vi "MSControl_main.vi"() -> ()   [LabVIEW 2017]
doc: "this is the start vi forMSControl program"
uses:
  Classes/StatusLog/StatusLog.lvclass
  Classes/PrepLineObject/PrepLineObject.lvclass
  Classes/Flags/flag.lvclass
  Classes/Plots/Plots.lvclass
  Classes/Standard/Standard.lvclass
  Classes/Spectrometer/Spectrometer.lvclass
  Classes/Analysis/Analysis.lvclass
  Classes/Instrument/instrument.lvclass
  Classes/MagFieldTable/MagFieldTable.lvclass
  Classes/Pipette/Pipette.lvclass
  Classes/Message/Message.lvclass
  global variables.vi
  <vilib>/Utility/config.llb/Read Key (U32).vi
  <vilib>/Utility/config.llb/Read Key (Path).vi
  <vilib>/Utility/config.llb/Read Key (String).vi
  <vilib>/Utility/config.llb/NI_LVConfig.lvlib
panel:
  in  "setup button":bool
  in  "start button":bool
  out "status string":string
  in  "error in (no error)":errorcluster
  out "error out":errorcluster
  # "MS Control"
  # "v20171231"
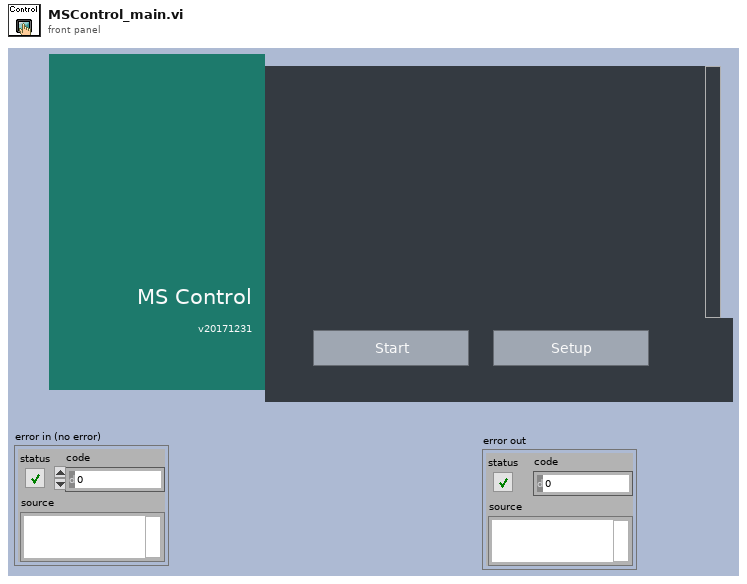
[diagram p1: front panel]
types:
  T1 = cluster{"log identifier":string, "active?":bool}[]
  T2 = cluster{"name":string, "inst-type":string, "class path":path, "class-name":string}[]
  T3 = cluster{"name":string, "class-name":string, "class path":path, "inst-type":string}
  T4 = cluster{"event name":enum16{"SwitchUpdate", "SysChkUpdate", "ScriptMessageUpdate"}}
  T5 = typedef "NI_LVConfig.lvlib/Config Data RefNum.ctl" = refnum<k1>
  T6 = cluster{"name":string, "class-name":string, "class path":path, "inst-type":string}[]
  T7 = cluster{"name":string, "inst-type":string, "class path":path, "class-name":string}
  T8 = typedef "Semaphore RefNum" = refnum<k1>
  T9 = enum32{"Invalid", "Standard", "Closed", "Hidden", "Minimized", "Maximized"}
  T10 = enum16{"Left Button", "Center Button", "Right Button", "Window Close"}
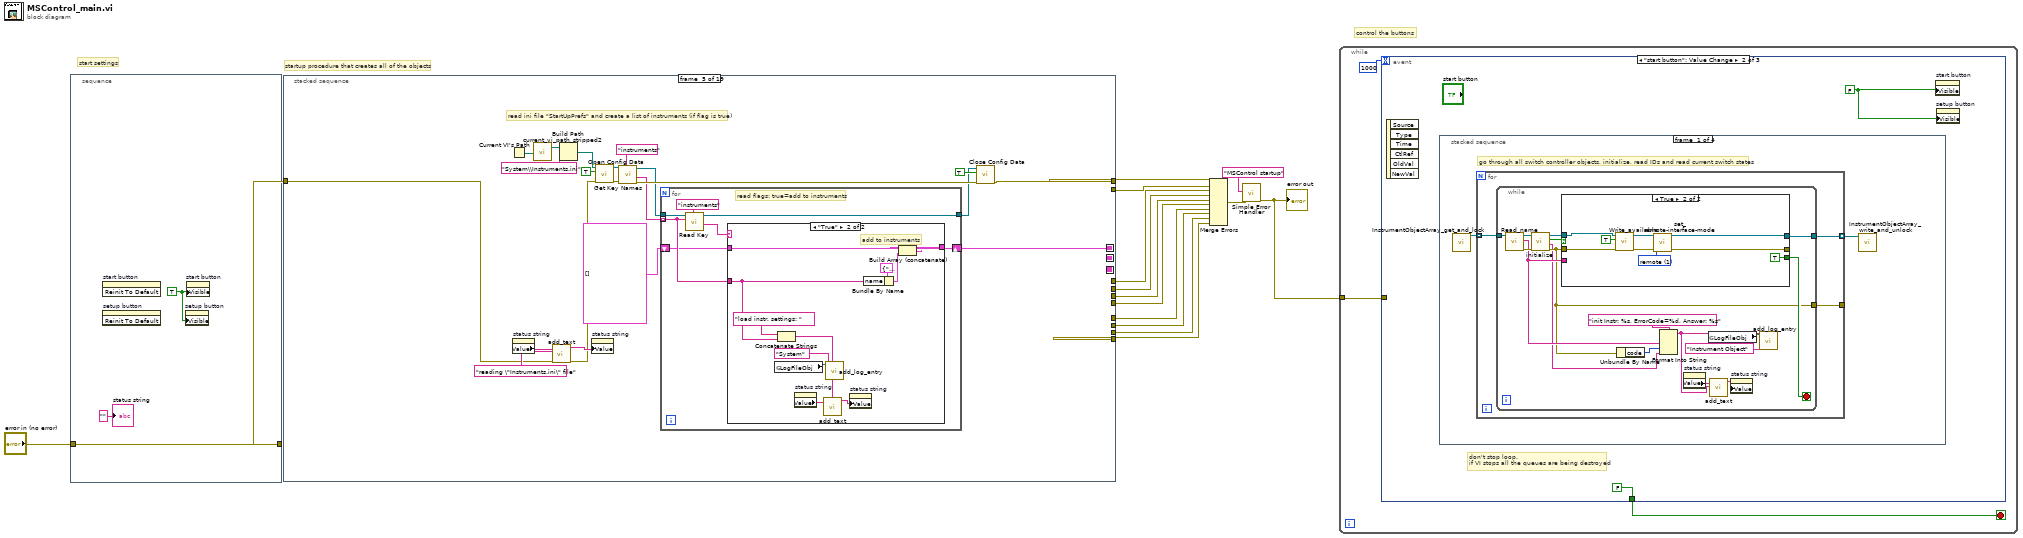
[diagram p0: block diagram]
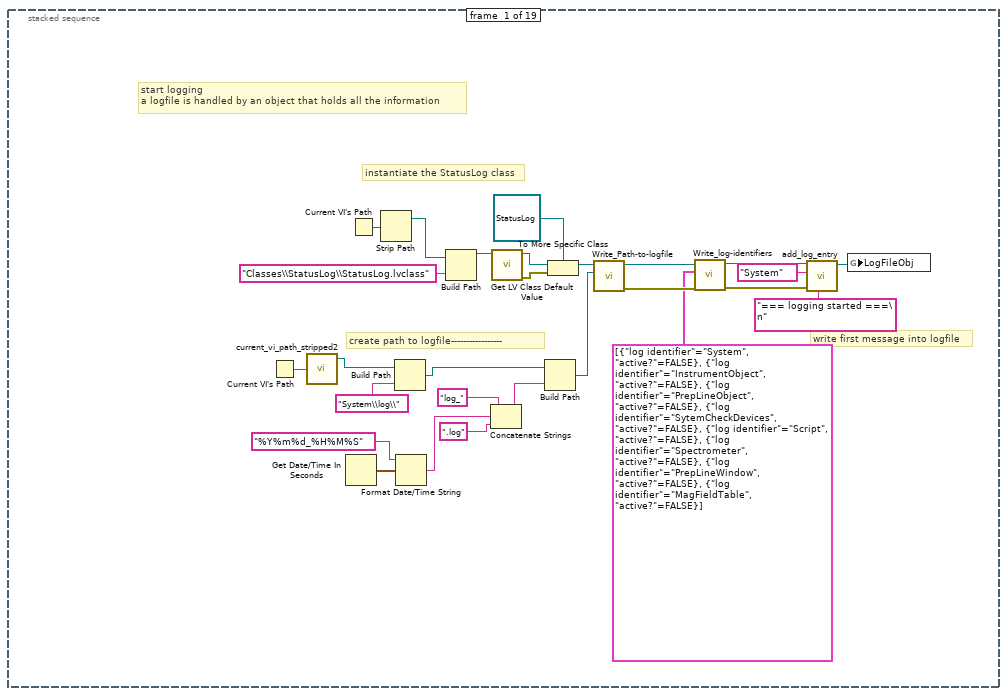
[diagram p2: hidden frame]
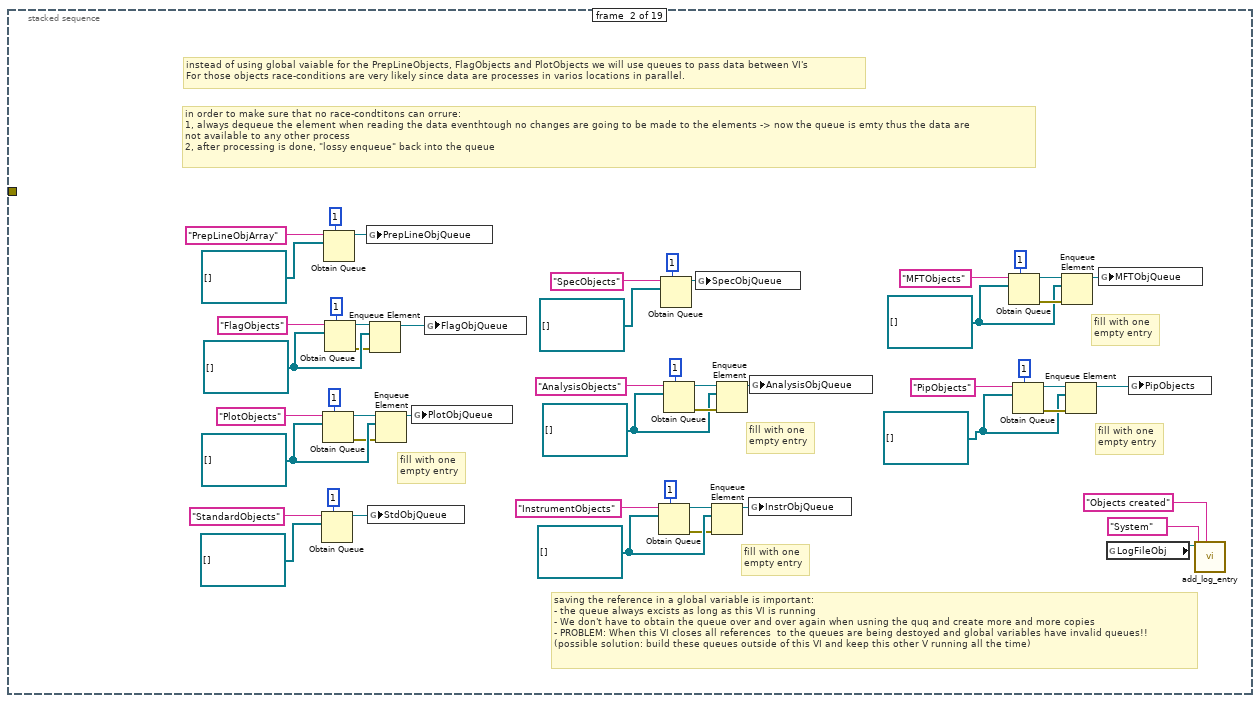
[diagram p3: hidden frame]
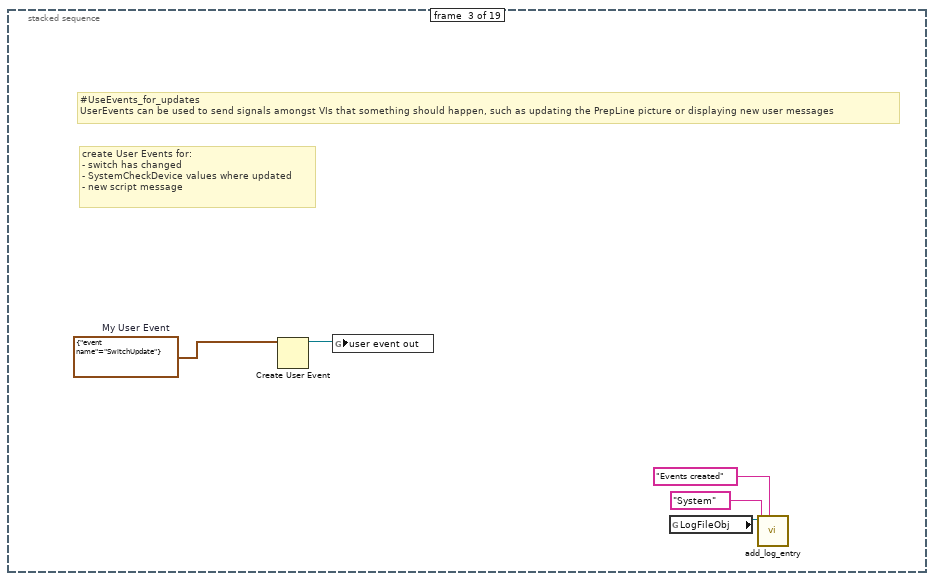
[diagram p4: hidden frame]
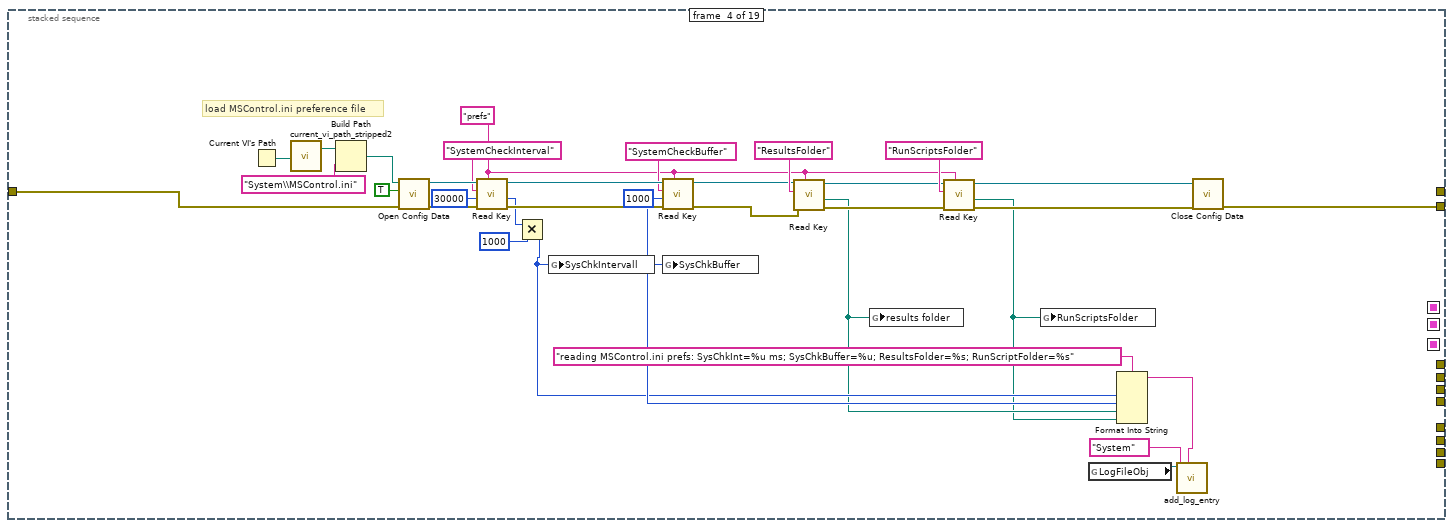
[diagram p5: hidden frame]
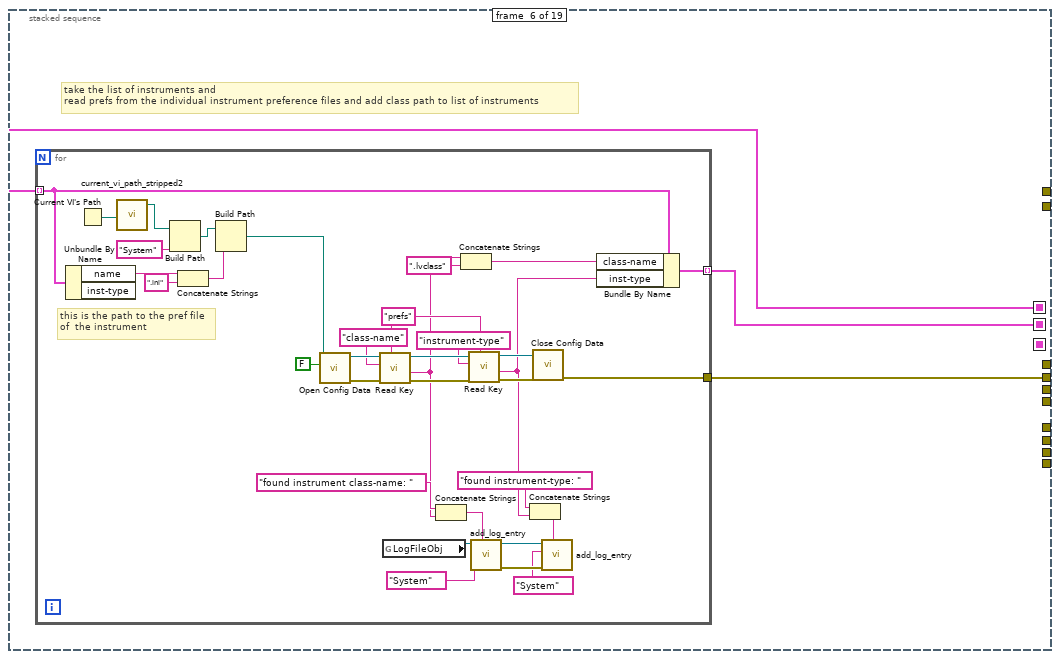
[diagram p7: hidden frame]
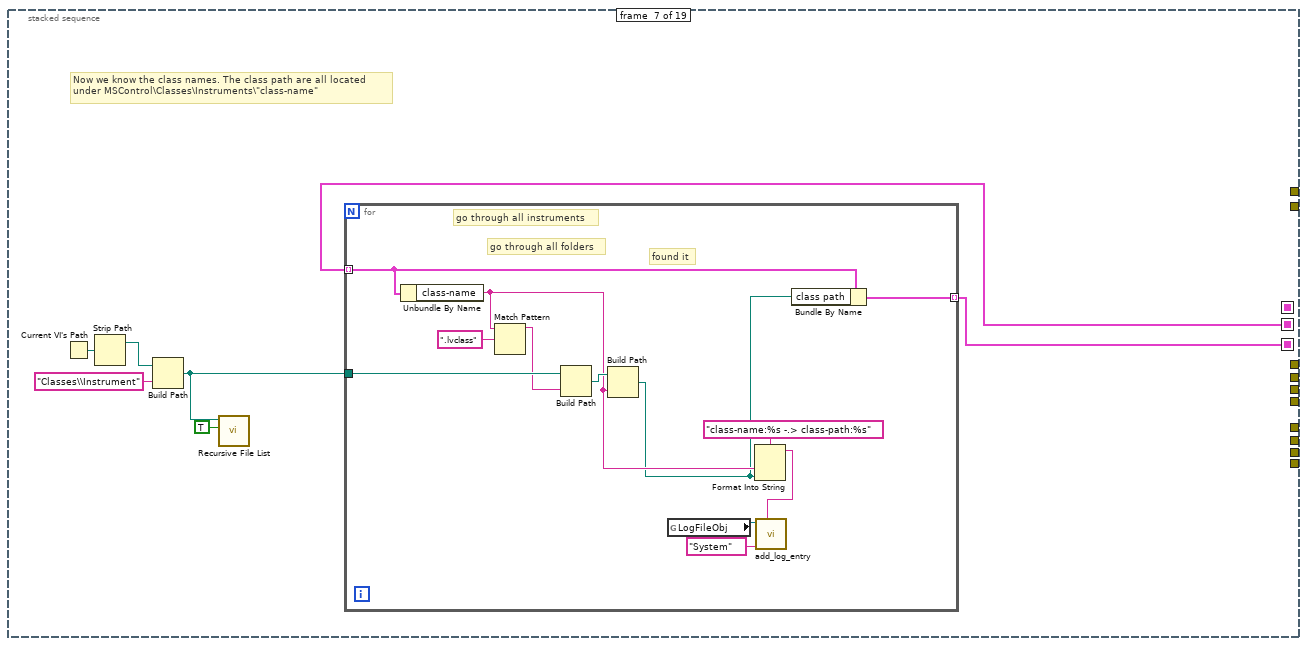
[diagram p8: hidden frame]
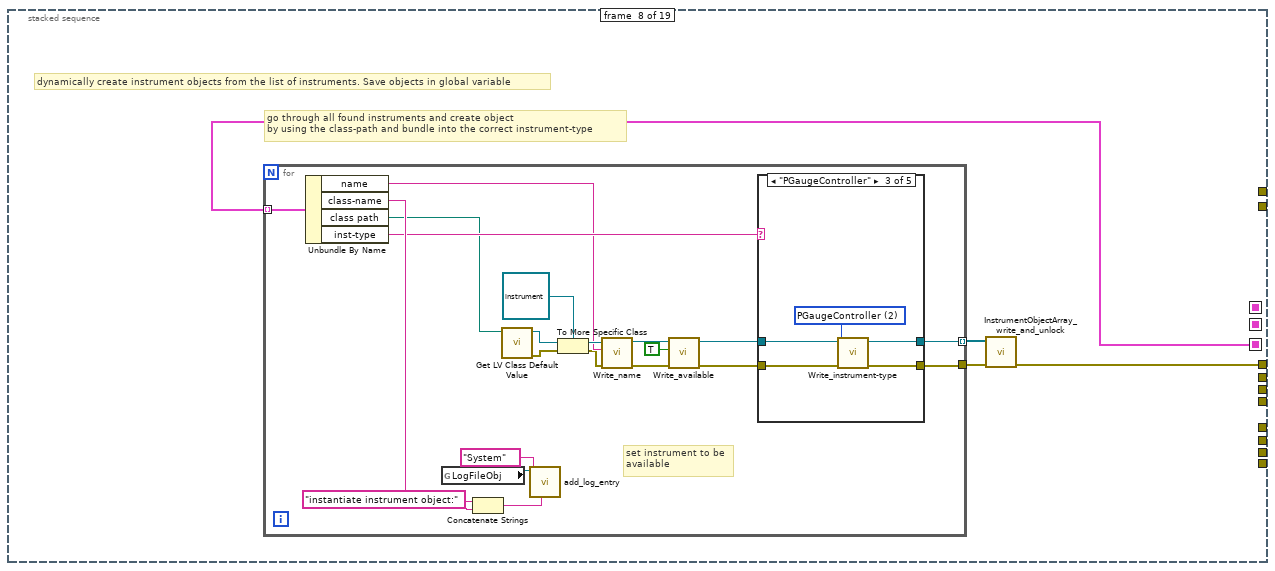
[diagram p9: hidden frame]
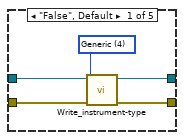
[diagram p10: hidden frame]
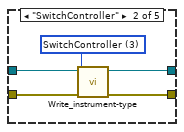
[diagram p11: hidden frame]
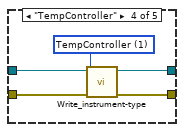
[diagram p12: hidden frame]
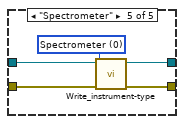
[diagram p13: hidden frame]
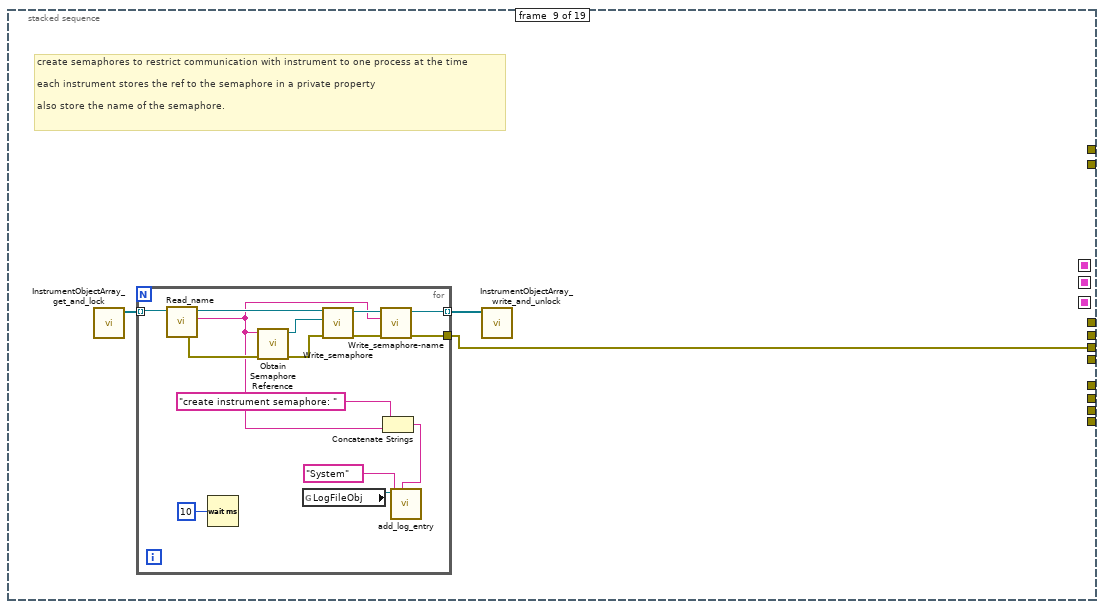
[diagram p14: hidden frame]
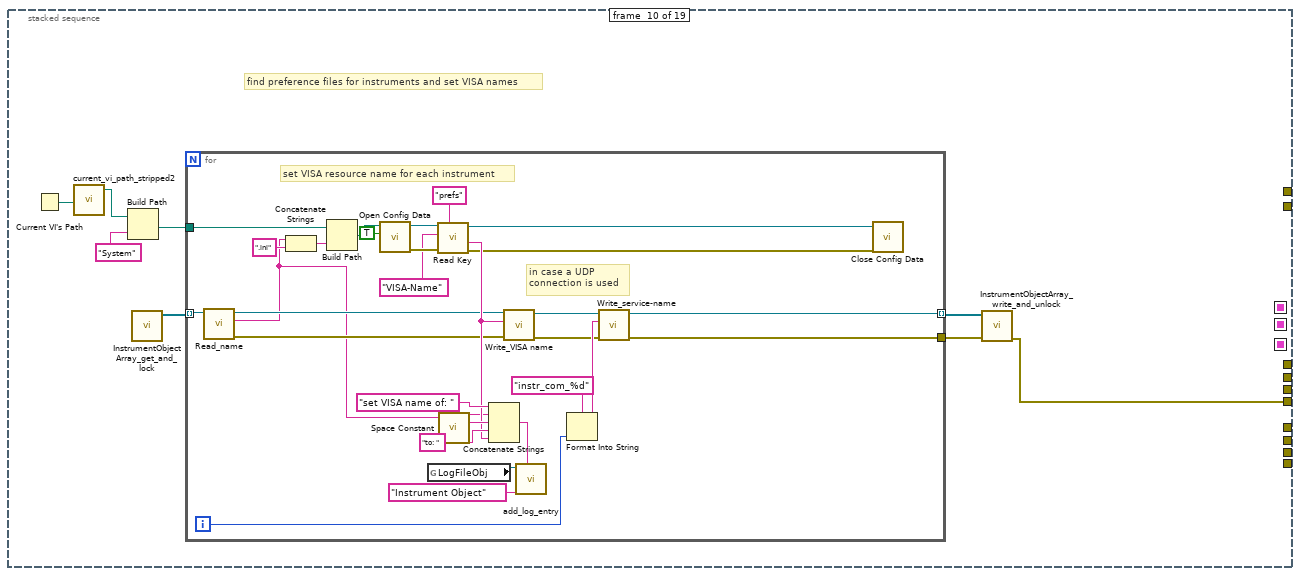
[diagram p15: hidden frame]
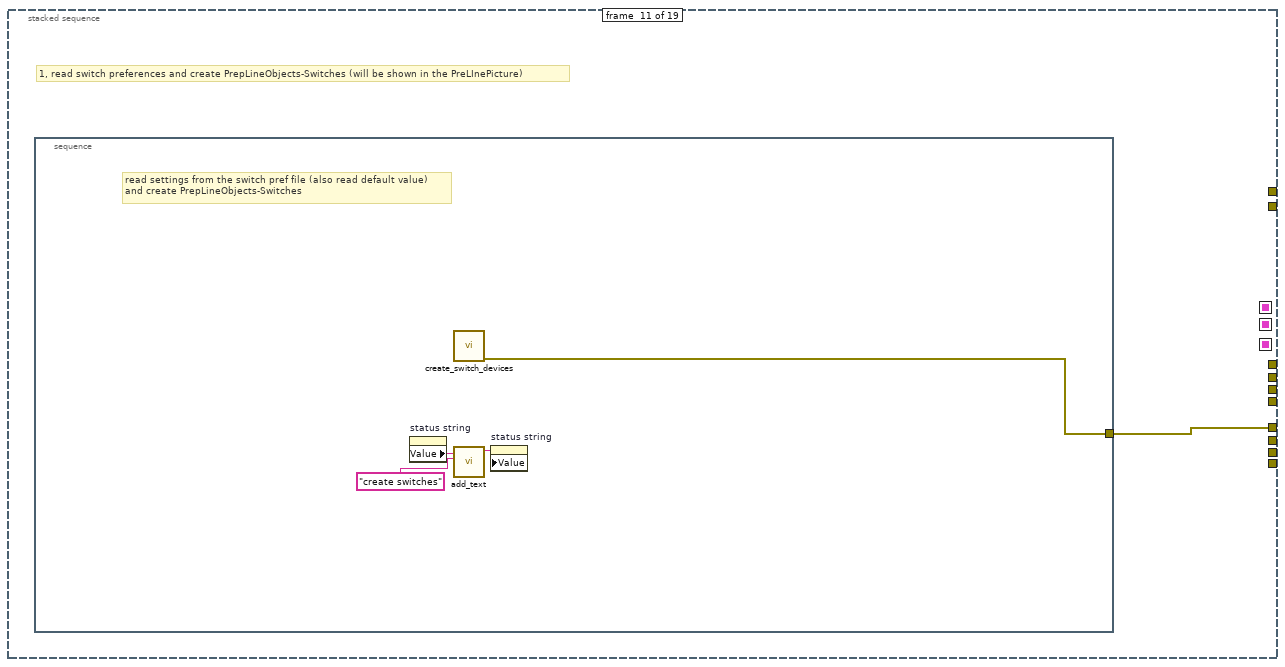
[diagram p16: hidden frame]
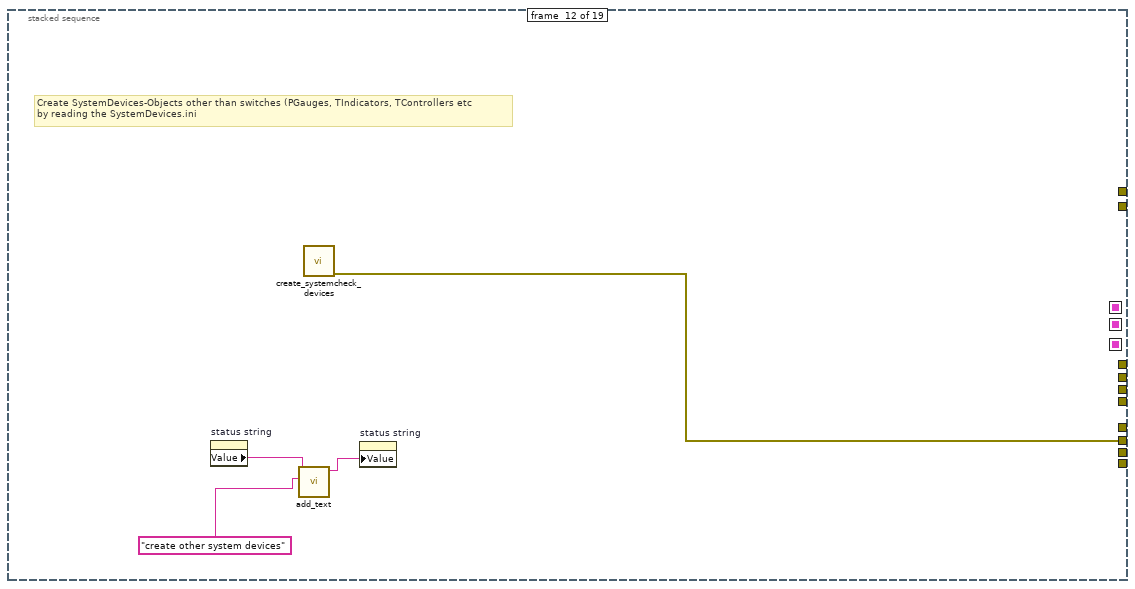
[diagram p17: hidden frame]
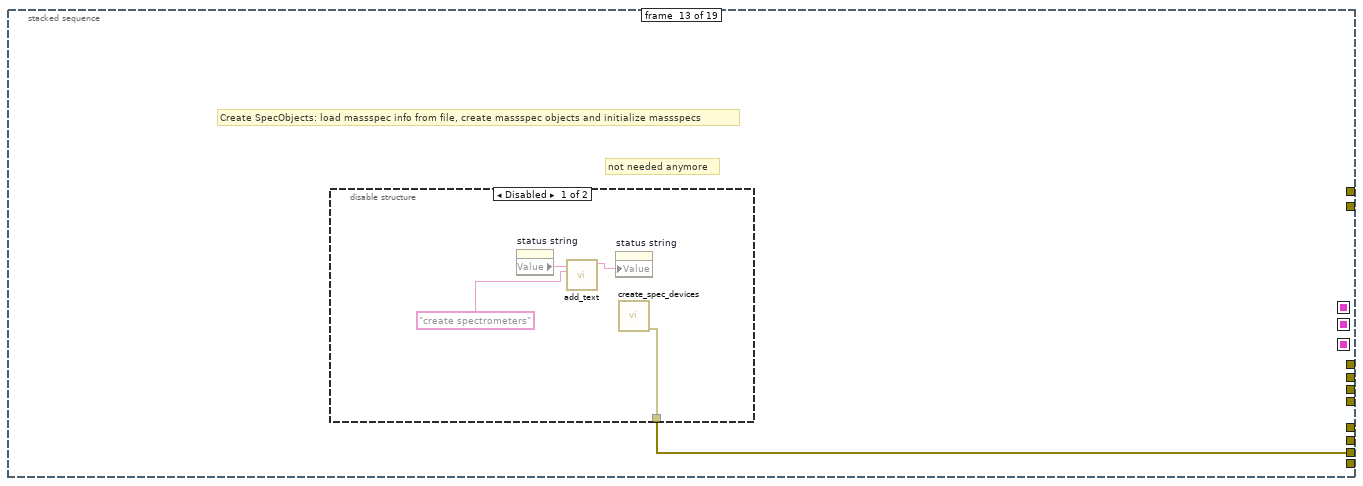
[diagram p18: hidden frame]
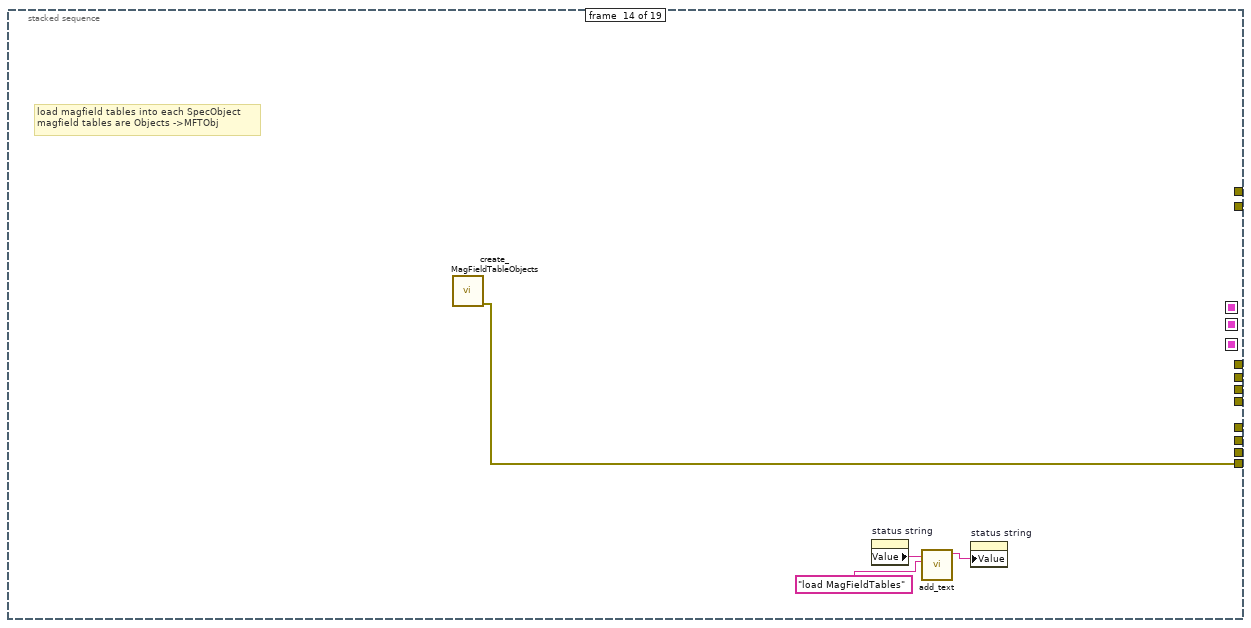
[diagram p20: hidden frame]
diagram:
  # "start settings"
  # "startup procedure that creates all of the objects"
  # "control the buttons"
  n1 = stacked-sequence {
    tunnel: [w17] -> w14
    tunnel: "error in (no error)" -> [w17]
    frame #0 {
      w16 = TRUE ("Visible")
      n2 = invoke on="start button" class="Bool (strict)" method="Reinit To Default"() -> ()  [unwired: 3 in, 3 out]
      n3 = invoke on="setup button" class="Bool (strict)" method="Reinit To Default"() -> ()  [unwired: 3 in, 3 out]
      n4 = property on="setup button" class="Bool (strict)"("Visible"=w16) -> ()  [unwired: 2 in, 2 out]
      n5 = property on="start button" class="Bool (strict)"("Visible"=w16) -> ()  [unwired: 2 in, 2 out]
      "status string" <- "" ("status string")
    }
  }
  n6 = stacked-sequence {
    seq-local: [_ _ _ _ w139 _ _ _ _ _ _ _ _ _ _ _ _ _ _] -> [_ _ _ _ _ w178 _ _ _ _ _ _ _ _ _ _ _ _ _]
    seq-local: [_ _ _ _ _ w177 _ _ _ _ _ _ _ _ _ _ _ _ _] -> [_ _ _ _ _ _ w218 _ _ _ _ _ _ _ _ _ _ _ _]
    seq-local: [_ _ _ _ _ _ w217 _ _ _ _ _ _ _ _ _ _ _ _] -> [_ _ _ _ _ _ _ w235 _ _ _ _ _ _ _ _ _ _ _]
    tunnel: w14 -> [_ _ _ w122 w141 _ _ _ _ _ _ _ _ _ _ _ _ _ _]
    tunnel: [_ _ _ _ w150 _ _ _ _ _ _ _ _ _ _ _ _ _ _] -> w13
    tunnel: [_ _ _ w121 _ _ _ _ _ _ _ _ _ _ _ _ _ _ _] -> w12
    tunnel: [_ _ _ _ _ w176 _ _ _ _ _ _ _ _ _ _ _ _ _] -> w10
    tunnel: [_ _ _ _ _ _ _ w232 _ _ _ _ _ _ _ _ _ _ _] -> w11
    tunnel: [_ _ _ _ _ _ _ _ w284 _ _ _ _ _ _ _ _ _ _] -> w9
    tunnel: [_ _ _ _ _ _ _ _ _ w300 _ _ _ _ _ _ _ _ _] -> w8
    tunnel: [_ _ _ _ _ _ _ _ _ _ w337 _ _ _ _ _ _ _ _] -> w7
    tunnel: [_ _ _ _ _ _ _ _ _ _ _ w345 _ _ _ _ _ _ _] -> w6
    tunnel: [_ _ _ _ _ _ _ _ _ _ _ _ w346 _ _ _ _ _ _] -> w3
    tunnel: [_ _ _ _ _ _ _ _ _ _ _ _ _ w351 _ _ _ _ _] -> w2
    frame #0 {
      # "write first message into logfile"
      # "create path to logfile-----------------"
      # "instantiate the StatusLog class"
      # "start logging\na logfile is handled by an object that holds all the information"
      n7 = Current VI's Path() -> (path=w20:path)
      n8 = call "current_vi_path_stripped2.vi"("current VI Path"=w20) -> ("current VI Path stripped out"=w19:path)  [unwired: 3 in, 1 out]
      n9 = Get Date/Time In Seconds() -> (seconds since 1Jan1904=w37:timestamp)
      n10 = Current VI's Path() -> (path=w22:path)
      n11 = Strip Path(path=w22) -> (stripped path=w21:path)  [unwired: 1 out]
      n12 = Build Path(base path=w19, name or relative path="System\\log\\") -> (appended path=w38:path)
      n13 = Format Date/Time String(time format string (%c)="%Y%m%d_%H%M%S", seconds (now)=w37) -> (date/time string=w33:string)  [unwired: 1 in]
      n14 = Build Path(base path=w21, name or relative path="Classes\\StatusLog\\StatusLog.lvclass") -> (appended path=w41:path)
      n15 = Concatenate Strings("log_" ("string"), w33, ".log" ("string")) -> (w35:string)
      n16 = call <vilib>:"Get LV Class Default Value.vi"("class path"=w41) -> ("error out"=w43:errorcluster, "object"=w44:refnum<class>)  [unwired: 1 in, 8 out]
      n17 = Build Path(base path=w38, name or relative path=w35) -> (appended path=w34:path)
      n18 = To More Specific Class(target class=refnum<class "StatusLog.lvclass"> refnum ("StatusLog.lvclass"), reference=w44, error in=w43) -> (specific class reference=w39:refnum<class "StatusLog.lvclass">)  [unwired: 1 out]
      n19 = call-dynamic "Write_Path-to-logfile.vi"("Path to logfile"=w34, "StatusLog in"=w39) -> ("error out"=w26:errorcluster, "StatusLog out"=w28:refnum<class "StatusLog.lvclass">)  [unwired: 8 in]
      n20 = call-dynamic "Write_log-identifiers.vi"("error in (no error)"=w26, "log identifiers"=T1 [{"log identifier"="System", "active?"=FALSE}, {"log identifier"="InstrumentObject", "active?"=FALSE}, {"log identifier"="PrepLineObject", "active?"=FALSE}, {"log identifier"="SytemCheckDevices", "active?"=FALSE}, {"log identifier"="Script", "active?"=FALSE}, {"log identifier"="Spectrometer", "active?"=FALSE}, {"log identifier"="PrepLineWindow", "active?"=FALSE}, {"log identifier"="MagFieldTable", "active?"=FALSE}], "StatusLog in"=w28) -> ("error out"=w25:errorcluster, "StatusLog out"=w27:refnum<class "StatusLog.lvclass">)  [unwired: 7 in]
      n21 = call-dynamic "add_log_entry.vi"("new entry"="=== logging started ===\n", "error in (no error)"=w25, "log identifiers"="System", "StatusLog in"=w27) -> ("StatusLog out"=w29:refnum<class "StatusLog.lvclass">)  [unwired: 4 in, 1 out]
      n22 = global write "global variables.vi" "LogFileObj"(w29) -> ()
    }
    frame #1 {
      w49 = refnum<class "Pipette.lvclass">[] [] ("PlotObjArray")
      w63 = refnum<class "MagFieldTable.lvclass">[] [] ("PlotObjArray")
      w66 = refnum<class "instrument.lvclass">[] [] ("PlotObjArray")
      w75 = refnum<class "Analysis.lvclass">[] [] ("PlotObjArray")
      w79 = refnum<class "Plots.lvclass">[] [] ("PlotObjArray")
      w57 = refnum<class "flag.lvclass">[] [] ("FlagObjArray")
      # "fill with one\nempty entry"
      # "fill with one\nempty entry"
      # "fill with one\nempty entry"
      # "fill with one\nempty entry"
      # "fill with one\nempty entry"
      # "saving the reference in a global variable is important:\n- the queue always excists as long as this VI is running\n- We don't have to obtain the queue over and over again when usning the quq and create more and more copies\n- PROBLEM: When this VI closes all references  to the queues are being destoyed and global variables have invalid queues!!\n(possible solution: build these queues outside of this VI and keep this other V running all the time)"
      # "in order to make sure that no race-condtitons can orrure:\n1, always dequeue the element when reading the data eventhtough no changes are going to be made to the elements -> now the queue is emty thus the data are\nnot available to any other process\n2, after processing is done, \"lossy enqueue\" back into the queue"
      # "instead of using global vaiable for the PrepLineObjects, FlagObjects and PlotObjects we will use queues to pass data between VI's\nFor those objects race-conditions are very likely since data are processes in varios locations in parallel."
      n23 = Obtain Queue(max queue size (-1, unlimited)=1, name (unnamed)="StandardObjects", element data type=refnum<class "Standard.lvclass">[] [] ("PlotObjArray")) -> (queue out=w85:refnum<queue>)  [unwired: 2 in, 2 out]
      n24 = Obtain Queue(max queue size (-1, unlimited)=1, name (unnamed)="PlotObjects", element data type=w79) -> (queue out=w80:refnum<queue>, error out=w77:errorcluster)  [unwired: 2 in, 1 out]
      n25 = Obtain Queue(max queue size (-1, unlimited)=1, name (unnamed)="PrepLineObjArray", element data type=refnum<class "PrepLineObject.lvclass">[] [] ("PrepLineObjArray")) -> (queue out=w89:refnum<queue>)  [unwired: 2 in, 2 out]
      n26 = Obtain Queue(max queue size (-1, unlimited)=1, name (unnamed)="FlagObjects", element data type=w57) -> (queue out=w58:refnum<queue>, error out=w56:errorcluster)  [unwired: 2 in, 1 out]
      n27 = global write "global variables.vi" "PrepLineObjQueue"(w89) -> ()
      n28 = global write "global variables.vi" "StdObjQueue"(w85) -> ()
      n29 = Enqueue Element(queue=w58, element=w57, error in (no error)=w56) -> (queue out=w55:refnum<queue>)  [unwired: 1 in, 2 out]
      n30 = Enqueue Element(queue=w80, element=w79, error in (no error)=w77) -> (queue out=w78:refnum<queue>)  [unwired: 1 in, 2 out]
      n31 = global write "global variables.vi" "PlotObjQueue"(w78) -> ()
      n32 = global write "global variables.vi" "FlagObjQueue"(w55) -> ()
      n33 = Obtain Queue(max queue size (-1, unlimited)=1, name (unnamed)="InstrumentObjects", element data type=w66) -> (queue out=w67:refnum<queue>, error out=w65:errorcluster)  [unwired: 2 in, 1 out]
      n34 = Obtain Queue(max queue size (-1, unlimited)=1, name (unnamed)="SpecObjects", element data type=refnum<class "Spectrometer.lvclass">[] [] ("PlotObjArray")) -> (queue out=w81:refnum<queue>)  [unwired: 2 in, 2 out]
      n35 = Obtain Queue(max queue size (-1, unlimited)=1, name (unnamed)="AnalysisObjects", element data type=w75) -> (queue out=w74:refnum<queue>, error out=w76:errorcluster)  [unwired: 2 in, 1 out]
      n36 = global write "global variables.vi" "SpecObjQueue"(w81) -> ()
      n37 = Enqueue Element(queue=w67, element=w66, error in (no error)=w65) -> (queue out=w70:refnum<queue>)  [unwired: 1 in, 2 out]
      n38 = Enqueue Element(queue=w74, element=w75, error in (no error)=w76) -> (queue out=w71:refnum<queue>)  [unwired: 1 in, 2 out]
      n39 = global write "global variables.vi" "InstrObjQueue"(w70) -> ()
      n40 = global write "global variables.vi" "AnalysisObjQueue"(w71) -> ()
      n41 = Obtain Queue(max queue size (-1, unlimited)=1, name (unnamed)="MFTObjects", element data type=w63) -> (queue out=w62:refnum<queue>, error out=w64:errorcluster)  [unwired: 2 in, 1 out]
      n42 = Obtain Queue(max queue size (-1, unlimited)=1, name (unnamed)="PipObjects", element data type=w49) -> (queue out=w51:refnum<queue>, error out=w50:errorcluster)  [unwired: 2 in, 1 out]
      n43 = Enqueue Element(queue=w62, element=w63, error in (no error)=w64) -> (queue out=w59:refnum<queue>)  [unwired: 1 in, 2 out]
      n44 = Enqueue Element(queue=w51, element=w49, error in (no error)=w50) -> (queue out=w54:refnum<queue>)  [unwired: 1 in, 2 out]
      n45 = global write "global variables.vi" "MFTObjQueue"(w59) -> ()
      n46 = global read "global variables.vi" "LogFileObj"() -> (w48:refnum<class "StatusLog.lvclass">)
      n47 = global write "global variables.vi" "PipObjects"(w54) -> ()
      n48 = call-dynamic "add_log_entry.vi"("new entry"="Objects created", "log identifiers"="System", "StatusLog in"=w48) -> ()  [unwired: 5 in, 2 out]
    }
    frame #2 {
      w101 = T4 {"event name"=enum."SwitchUpdate"}  # My User Event
      # "#UseEvents_for_updates\nUserEvents can be used to send signals amongst VIs that something should happen, such as updating the PrepLine picture or displaying new user messages"
      # "create User Events for:\n- switch has changed\n- SystemCheckDevice values where updated\n- new script message"
      n49 = Create User Event(user event datatype=w101) -> (user event=w100:refnum<user-event>)  [unwired: 1 in, 1 out]
      n50 = global write "global variables.vi" "user event out"(w100) -> ()
      n51 = global read "global variables.vi" "LogFileObj"() -> (w99:refnum<class "StatusLog.lvclass">)
      n52 = call-dynamic "add_log_entry.vi"("new entry"="Events created", "log identifiers"="System", "StatusLog in"=w99) -> ()  [unwired: 5 in, 2 out]
    }
    frame #3 {
      w105 = "prefs" ("section")
      # "load MSControl.ini preference file"
      n53 = Current VI's Path() -> (path=w132:path)
      n54 = call "current_vi_path_stripped2.vi"("current VI Path"=w132) -> ("current VI Path stripped out"=w131:path)  [unwired: 3 in, 1 out]
      n55 = Build Path(base path=w131, name or relative path="System\\MSControl.ini") -> (appended path=w133:path)
      n56 = call <vilib>:"Open Config Data.vi"("error in (no error)"=w122, "create file if necessary (T)"=TRUE, "configuration file path"=w133) -> ("error out"=w130:errorcluster, "refnum"=w129:T5)  [unwired: 6 in, 1 out]
      n57 = call-poly <vilib>:"Read Key.vi"("section"=w105, "error in (no error)"=w130, "default value"=u32 30000, "key"="SystemCheckInterval" ("section"), "refnum"=w129) -> ("error out"=w127:errorcluster, "value"=w116:u32, "refnum out"=w128:T5)  [unwired: 3 in, 1 out]
      n58 = Multiply(x=w116, y=u32 1000) -> (x*y=w114:u32)
      n59 = global write "global variables.vi" "SysChkIntervall"(w114) -> ()
      n60 = call-poly <vilib>:"Read Key.vi"("section"=w105, "error in (no error)"=w127, "default value"=u32 1000, "key"="SystemCheckBuffer" ("section"), "refnum"=w128) -> ("error out"=w111:errorcluster, "value"=w117:u32, "refnum out"=w112:T5)  [unwired: 3 in, 1 out]
      n61 = global write "global variables.vi" "SysChkBuffer"(w117) -> ()
      n62 = call-poly <vilib>:"Read Key.vi"("section"=w105, "error in (no error)"=w111, "key"="ResultsFolder" ("section"), "refnum"=w112) -> ("error out"=w108:errorcluster, "value"=w104:path, "refnum out"=w109:T5)  [unwired: 4 in, 1 out]
      n63 = global write "global variables.vi" "results folder"(w104) -> ()
      n64 = call-poly <vilib>:"Read Key.vi"("section"=w105, "error in (no error)"=w108, "key"="RunScriptsFolder" ("section"), "refnum"=w109) -> ("error out"=w106:errorcluster, "value"=w103:path, "refnum out"=w107:T5)  [unwired: 4 in, 1 out]
      n65 = global write "global variables.vi" "RunScriptsFolder"(w103) -> ()
      n66 = global read "global variables.vi" "LogFileObj"() -> (w120:refnum<class "StatusLog.lvclass">)
      n67 = Format Into String(format string="reading MSControl.ini prefs: SysChkInt=%u ms; SysChkBuffer=%u; ResultsFolder=%s; RunScriptFolder=%s", w114, w117, w104, w103) -> (resulting string=w102:string)  [unwired: 2 in, 1 out]
      n68 = call-dynamic "add_log_entry.vi"("new entry"=w102, "log identifiers"="System", "StatusLog in"=w120) -> ()  [unwired: 5 in, 2 out]
      n69 = call <vilib>:"Close Config Data.vi"("error in (no error)"=w106, "refnum"=w107) -> ("error out"=w121:errorcluster)  [unwired: 8 in, 1 out]
    }
    frame #4 {
      # "read ini file \"StartUpPrefs\" and create a list of instruments (if flag is true)"
      n70 = Current VI's Path() -> (path=w137:path)
      n71 = property on="status string" class="Str"() -> ("Value"=w144:string)  [unwired: 2 in, 2 out]
      n72 = call "current_vi_path_stripped2.vi"("current VI Path"=w137) -> ("current VI Path stripped out"=w136:path)  [unwired: 3 in, 1 out]
      n73 = call "add_text.vi"("error in (no error)"=w141, "string in"="reading \"Instruments.ini\" file" ("string"), "new string"=w144) -> ("error out"=w140:errorcluster, "string out"=w142:string)  [unwired: 7 in]
      n74 = Build Path(base path=w136, name or relative path="System\\Instruments.ini") -> (appended path=w148:path)
      n75 = property on="status string" class="Str"("Value"=w142) -> ()  [unwired: 2 in, 2 out]
      n76 = call <vilib>:"Open Config Data.vi"("error in (no error)"=w140, "create file if necessary (T)"=TRUE, "configuration file path"=w148) -> ("error out"=w153:errorcluster, "refnum"=w154:T5)  [unwired: 6 in, 1 out]
      n77 = call <vilib>:"Get Key Names.vi"("section"="instruments", "error in (no error)"=w153, "refnum"=w154) -> ("error out"=w151:errorcluster, "key names"=w147:string[], "refnum out"=w146:T5)  [unwired: 5 in, 1 out]
      n78 = for {
        tunnel: w147 -> [w160] mode=indexing
        tunnel: w146 -> [w163]
        tunnel: [w162] -> w145
        shift-right: [w157] -> w139
        shift-left: T2 [] -> [w158]
        # "read flags: true=add to instruments"
        n79 = call-poly <vilib>:"Read Key.vi"("section"="instruments", "key"=w160, "refnum"=w163) -> ("value"=w159:string, "refnum out"=w162:T5)  [unwired: 5 in, 2 out]
        n80 = case shown="\"True\"" w159 {
          tunnel: w160 -> [_ w168]
          tunnel: [w164 w173] -> w157
          tunnel: w158 -> [w164 w175]
          frame "False", Default {
            # "don't add to instruments\nbecause it's set to false"
          }
          frame "True" {
            # "add to instruments"
            n81 = global read "global variables.vi" "LogFileObj"() -> (w167:refnum<class "StatusLog.lvclass">)
            n82 = Concatenate Strings("load instr. settings: " ("string"), w168) -> (w165:string)
            n83 = property on="status string" class="Str"() -> ("Value"=w170:string)  [unwired: 2 in, 2 out]
            n84 = call "add_text.vi"("string in"=w165, "new string"=w170) -> ("string out"=w171:string)  [unwired: 8 in, 1 out]
            n85 = call-dynamic "add_log_entry.vi"("new entry"=w165, "log identifiers"="System", "StatusLog in"=w167) -> ()  [unwired: 5 in, 2 out]
            n86 = property on="status string" class="Str"("Value"=w171) -> ()  [unwired: 2 in, 2 out]
            n87 = Bundle By Name(cluster=T3 {"name"="", "class-name"="", "class path"=path "", "inst-type"=""}, "name"=w168) -> (w174:T3)
            n88 = Build Array (concatenate)(w175, w174) -> (w173:T6)
          }
        }
      }
      n89 = call <vilib>:"Close Config Data.vi"("error in (no error)"=w151, "write file if changed (T)"=TRUE, "refnum"=w145) -> ("error out"=w150:errorcluster)  [unwired: 7 in, 1 out]
    }
    frame #5 {
      # "take the list of instruments and\nread prefs from the individual instrument preference files and add class path to list of instruments"
      n90 = for {
        tunnel: w178 -> [w202] mode=indexing
        tunnel: [w201] -> w177 mode=indexing
        tunnel: [w179] -> w176
        w196 = "prefs" ("section")
        # "this is the path to the pref file\nof  the instrument"
        n91 = Unbundle By Name(w202) -> ("name"=w205:string)  [unwired: 1 out]
        n92 = Current VI's Path() -> (path=w181:path)
        n93 = call "current_vi_path_stripped2.vi"("current VI Path"=w181) -> ("current VI Path stripped out"=w180:path)  [unwired: 3 in, 1 out]
        n94 = Build Path(base path=w180, name or relative path="System") -> (appended path=w210:path)
        n95 = Concatenate Strings(w205, ".ini" ("string")) -> (w203:string)
        n96 = Build Path(base path=w210, name or relative path=w203) -> (appended path=w209:path)
        n97 = call <vilib>:"Open Config Data.vi"("create file if necessary (T)"=FALSE, "configuration file path"=w209) -> ("error out"=w208:errorcluster, "refnum"=w207:T5)  [unwired: 7 in, 1 out]
        n98 = call-poly <vilib>:"Read Key.vi"("section"=w196, "error in (no error)"=w208, "key"="class-name", "refnum"=w207) -> ("error out"=w198:errorcluster, "value"=w183:string, "refnum out"=w200:T5)  [unwired: 4 in, 1 out]
        n99 = global read "global variables.vi" "LogFileObj"() -> (w193:refnum<class "StatusLog.lvclass">)
        n100 = Concatenate Strings("found instrument class-name: " ("string"), w183) -> (w192:string)
        n101 = Concatenate Strings(w183, ".lvclass" ("string")) -> (w184:string)
        n102 = call-poly <vilib>:"Read Key.vi"("section"=w196, "error in (no error)"=w198, "key"="instrument-type", "refnum"=w200) -> ("error out"=w197:errorcluster, "value"=w187:string, "refnum out"=w199:T5)  [unwired: 4 in, 1 out]
        n103 = call-dynamic "add_log_entry.vi"("new entry"=w192, "log identifiers"="System", "StatusLog in"=w193) -> ("error out"=w190:errorcluster, "StatusLog out"=w191:refnum<class "StatusLog.lvclass">)  [unwired: 5 in]
        n104 = Concatenate Strings("found instrument-type: " ("string"), w187) -> (w189:string)
        n105 = call <vilib>:"Close Config Data.vi"("error in (no error)"=w197, "refnum"=w199) -> ("error out"=w179:errorcluster)  [unwired: 8 in, 1 out]
        n106 = call-dynamic "add_log_entry.vi"("new entry"=w189, "error in (no error)"=w190, "log identifiers"="System", "StatusLog in"=w191) -> ()  [unwired: 4 in, 2 out]
        n107 = Bundle By Name(cluster=w202, "class-name"=w184, "inst-type"=w187) -> (w201:T7)
      }
    }
    frame #6 {
      # "Now we know the class names. The class path are all located\nunder MSControl\\Classes\\Instruments\\\"class-name\""
      n108 = Current VI's Path() -> (path=w216:path)
      n109 = Strip Path(path=w216) -> (stripped path=w215:path)  [unwired: 1 out]
      n110 = Build Path(base path=w215, name or relative path="Classes\\Instrument") -> (appended path=w213:path)
      n111 = call <vilib>:"Recursive File List.vi"("Treat LLBs as Folders?"=TRUE, "Folder Path"=w213) -> ()  [unwired: 5 in, 5 out]
      n112 = for {
        tunnel: w218 -> [w230] mode=indexing
        tunnel: w213 -> [w224]
        tunnel: [w231] -> w217 mode=indexing
        # "found it"
        # "go through all folders"
        # "go through all instruments"
        n113 = Unbundle By Name(w230) -> ("class-name"=w221:string)
        n114 = Match Pattern(string=w221, regular expression=".lvclass" ("string")) -> (before substring=w223:string)  [unwired: 1 in, 3 out]
        n115 = Build Path(base path=w224, name or relative path=w223) -> (appended path=w222:path)
        n116 = Build Path(base path=w222, name or relative path=w221) -> (appended path=w220:path)
        n117 = global read "global variables.vi" "LogFileObj"() -> (w229:refnum<class "StatusLog.lvclass">)
        n118 = Format Into String(format string="class-name:%s -.> class-path:%s", w221, w220) -> (resulting string=w227:string)  [unwired: 2 in, 1 out]
        n119 = call-dynamic "add_log_entry.vi"("new entry"=w227, "log identifiers"="System", "StatusLog in"=w229) -> ()  [unwired: 5 in, 2 out]
        n120 = Bundle By Name(cluster=w230, "class path"=w220) -> (w231:T7)
      }
    }
    frame #7 {
      # "go through all found instruments and create object\nby using the class-path and bundle into the correct instrument-type"
      # "dynamically create instrument objects from the list of instruments. Save objects in global variable"
      n121 = for {
        tunnel: w235 -> [w256] mode=indexing
        tunnel: [w253] -> w234 mode=indexing
        tunnel: [w241] -> w233
        # "set instrument to be\navailable"
        n122 = Unbundle By Name(w256) -> ("name"=w244:string, "class-name"=w255:string, "class path"=w243:path, "inst-type"=w254:string)
        n123 = global read "global variables.vi" "LogFileObj"() -> (w251:refnum<class "StatusLog.lvclass">)
        n124 = Concatenate Strings("instantiate instrument object:" ("string"), w255) -> (w250:string)
        n125 = call <vilib>:"Get LV Class Default Value.vi"("class path"=w243) -> ("error out"=w247:errorcluster, "object"=w248:refnum<class>)  [unwired: 1 in, 8 out]
        n126 = call-dynamic "add_log_entry.vi"("new entry"=w250, "log identifiers"="System", "StatusLog in"=w251) -> ()  [unwired: 5 in, 2 out]
        n127 = To More Specific Class(target class=refnum<class "instrument.lvclass"> refnum ("instrument.lvclass"), reference=w248, error in=w247) -> (specific class reference=w246:refnum<class "instrument.lvclass">, error out=w242:errorcluster)
        n128 = call-dynamic "Write_name.vi"("error in (no error)"=w242, "name"=w244, "instrument in"=w246) -> ("error out"=w239:errorcluster, "instrument out"=w240:refnum<class "instrument.lvclass">)  [unwired: 7 in]
        n129 = call-dynamic "Write_available.vi"("error in (no error)"=w239, "available?"=TRUE, "instrument in"=w240) -> ("error out"=w237:errorcluster, "instrument out"=w238:refnum<class "instrument.lvclass">)  [unwired: 7 in]
        n130 = case shown="\"PGaugeController\"" w254 {
          tunnel: [w261 w265 w270 w275 w280] -> w253
          tunnel: w238 -> [w260 w264 w269 w274 w279]
          tunnel: w237 -> [w259 w263 w268 w273 w278]
          tunnel: [w258 w262 w267 w272 w277] -> w241
          frame "False", Default {
            w257 = u16 4 items=["Spectrometer", "TempController", "PGaugeController", "SwitchController", "Generic"] ("instrument type")
            n131 = call-dynamic "Write_instrument-type.vi"("error in (no error)"=w259, "instrument type"=w257, "instrument in"=w260) -> ("error out"=w258:errorcluster, "instrument out"=w261:refnum<class "instrument.lvclass">)  [unwired: 7 in]
          }
          frame "SwitchController" {
            w266 = u16 3 items=["Spectrometer", "TempController", "PGaugeController", "SwitchController"] ("instrument type")
            n132 = call-dynamic "Write_instrument-type.vi"("error in (no error)"=w263, "instrument type"=w266, "instrument in"=w264) -> ("error out"=w262:errorcluster, "instrument out"=w265:refnum<class "instrument.lvclass">)  [unwired: 7 in]
          }
          frame "PGaugeController" {
            w271 = u16 2 items=["Spectrometer", "TempController", "PGaugeController", "SwitchController"] ("instrument type")
            n133 = call-dynamic "Write_instrument-type.vi"("error in (no error)"=w268, "instrument type"=w271, "instrument in"=w269) -> ("error out"=w267:errorcluster, "instrument out"=w270:refnum<class "instrument.lvclass">)  [unwired: 7 in]
          }
          frame "TempController" {
            w276 = u16 1 items=["Spectrometer", "TempController", "PGaugeController", "SwitchController"] ("instrument type")
            n134 = call-dynamic "Write_instrument-type.vi"("error in (no error)"=w273, "instrument type"=w276, "instrument in"=w274) -> ("error out"=w272:errorcluster, "instrument out"=w275:refnum<class "instrument.lvclass">)  [unwired: 7 in]
          }
          frame "Spectrometer" {
            w281 = u16 0 items=["Spectrometer", "TempController", "PGaugeController", "SwitchController"] ("instrument type")
            n135 = call-dynamic "Write_instrument-type.vi"("error in (no error)"=w278, "instrument type"=w281, "instrument in"=w279) -> ("error out"=w277:errorcluster, "instrument out"=w280:refnum<class "instrument.lvclass">)  [unwired: 7 in]
          }
        }
      }
      n136 = call "InstrumentObjectArray_write_and_unlock.vi"("error in (no error)"=w233, "InstrumentObjects"=w234) -> ("error out"=w232:errorcluster)  [unwired: 9 in]
    }
    frame #8 {
      # "create semaphores to restrict communication with instrument to one process at the time\n\neach instrument stores the ref to the semaphore in a private property\n\nalso store the name of the semaphore."
      n137 = call "InstrumentObjectArray_get_and_lock.vi"() -> ("InstrumentsObjects"=w283:refnum<class "instrument.lvclass">[])  [unwired: 10 in, 1 out]
      n138 = for {
        tunnel: w283 -> [w299] mode=indexing
        tunnel: [w292] -> w282 mode=indexing
        tunnel: [w291] -> w284
        n139 = call-dynamic "Read_name.vi"("instrument in"=w299) -> ("error out"=w298:errorcluster, "name"=w287:string, "instrument out"=w296:refnum<class "instrument.lvclass">)  [unwired: 8 in]
        n140 = Wait (ms)(milliseconds to wait=u32 10) -> ()  [unwired: 1 out]
        n141 = call <vilib>:"Obtain Semaphore Reference.vi"("error in (no error)"=w298, "name (unnamed)"=w287) -> ("error out"=w295:errorcluster, "semaphore"=w297:T8)  [unwired: 3 in, 1 out]
        n142 = global read "global variables.vi" "LogFileObj"() -> (w289:refnum<class "StatusLog.lvclass">)
        n143 = call-dynamic "Write_semaphore.vi"("error in (no error)"=w295, "semaphore"=w297, "instrument in"=w296) -> ("error out"=w293:errorcluster, "instrument out"=w294:refnum<class "instrument.lvclass">)  [unwired: 7 in]
        n144 = call-dynamic "Write_semaphore-name.vi"("error in (no error)"=w293, "semaphore name"=w287, "instrument in"=w294) -> ("error out"=w291:errorcluster, "instrument out"=w292:refnum<class "instrument.lvclass">)  [unwired: 7 in]
        n145 = Concatenate Strings("create instrument semaphore: " ("new entry"), w287) -> (w286:string)
        n146 = call-dynamic "add_log_entry.vi"("new entry"=w286, "log identifiers"="System", "StatusLog in"=w289) -> ()  [unwired: 5 in, 2 out]
      }
      n147 = call "InstrumentObjectArray_write_and_unlock.vi"("InstrumentObjects"=w282) -> ()  [unwired: 10 in, 1 out]
    }
    frame #9 {
      # "find preference files for instruments and set VISA names"
      n148 = Current VI's Path() -> (path=w305:path)
      n149 = call "current_vi_path_stripped2.vi"("current VI Path"=w305) -> ("current VI Path stripped out"=w304:path)  [unwired: 3 in, 1 out]
      n150 = Build Path(base path=w304, name or relative path="System") -> (appended path=w306:path)
      n151 = call "InstrumentObjectArray_get_and_lock.vi"() -> ("InstrumentsObjects"=w303:refnum<class "instrument.lvclass">[])  [unwired: 10 in, 1 out]
      n152 = for {
        tunnel: w306 -> [w336]
        tunnel: w303 -> [w324] mode=indexing
        tunnel: [w315] -> w302 mode=indexing
        tunnel: [w311] -> w301
        i -> [w313]
        # "in case a UDP\nconnection is used"
        # "set VISA resource name for each instrument"
        n153 = call-dynamic "Read_name.vi"("instrument in"=w324) -> ("error out"=w322:errorcluster, "name"=w321:string, "instrument out"=w323:refnum<class "instrument.lvclass">)  [unwired: 8 in]
        n154 = Concatenate Strings(w321, ".ini" ("string")) -> (w335:string)
        n155 = Build Path(base path=w336, name or relative path=w335) -> (appended path=w328:path)
        n156 = call <vilib>:"Open Config Data.vi"("create file if necessary (T)"=TRUE, "configuration file path"=w328) -> ("error out"=w332:errorcluster, "refnum"=w331:T5)  [unwired: 7 in, 1 out]
        n157 = global read "global variables.vi" "LogFileObj"() -> (w320:refnum<class "StatusLog.lvclass">)
        n158 = call-poly <vilib>:"Read Key.vi"("section"="prefs", "error in (no error)"=w332, "key"="VISA-Name", "refnum"=w331) -> ("error out"=w308:errorcluster, "value"=w325:string, "refnum out"=w309:T5)  [unwired: 4 in, 1 out]
        n159 = call <vilib>:"Space Constant.vi"() -> ("String"=w327:string)
        n160 = Concatenate Strings("set VISA name of: " ("string"), w321, w327, "to: " ("string"), w325) -> (w319:string)
        n161 = call-dynamic "Write_VISA name.vi"("error in (no error)"=w322, "VISA resource name"=w325, "instrument in"=w323) -> ("error out"=w314:errorcluster, "instrument out"=w316:refnum<class "instrument.lvclass">)  [unwired: 7 in]
        n162 = call-dynamic "add_log_entry.vi"("new entry"=w319, "log identifiers"="Instrument Object", "StatusLog in"=w320) -> ()  [unwired: 5 in, 2 out]
        n163 = Format Into String(format string="instr_com_%d" ("service name"), w313) -> (resulting string=w317:string)  [unwired: 2 in, 1 out]
        n164 = call-dynamic "Write_service-name.vi"("error in (no error)"=w314, "service name"=w317, "instrument in"=w316) -> ("error out"=w311:errorcluster, "instrument out"=w315:refnum<class "instrument.lvclass">)  [unwired: 7 in]
        n165 = call <vilib>:"Close Config Data.vi"("error in (no error)"=w308, "refnum"=w309) -> ()  [unwired: 8 in, 2 out]
      }
      n166 = call "InstrumentObjectArray_write_and_unlock.vi"("error in (no error)"=w301, "InstrumentObjects"=w302) -> ("error out"=w300:errorcluster)  [unwired: 9 in]
    }
    frame #10 {
      # "1, read switch preferences and create PrepLineObjects-Switches (will be shown in the PreLInePicture)"
      n167 = stacked-sequence {
        tunnel: [w338] -> w337
        frame #0 {
          # "read settings from the switch pref file (also read default value)\nand create PrepLineObjects-Switches"
          n168 = property on="status string" class="Str"() -> ("Value"=w340:string)  [unwired: 2 in, 2 out]
          n169 = call "create_switch_devices.vi"() -> ("error out"=w338:errorcluster)  [unwired: 11 in]
          n170 = call "add_text.vi"("string in"="create switches", "new string"=w340) -> ("string out"=w339:string)  [unwired: 8 in, 1 out]
          n171 = property on="status string" class="Str"("Value"=w339) -> ()  [unwired: 2 in, 2 out]
        }
      }
    }
    frame #11 {
      # "Create SystemDevices-Objects other than switches (PGauges, TIndicators, TControllers etc\nby reading the SystemDevices.ini"
      n172 = property on="status string" class="Str"() -> ("Value"=w343:string)  [unwired: 2 in, 2 out]
      n173 = call "add_text.vi"("string in"="create other system devices", "new string"=w343) -> ("string out"=w342:string)  [unwired: 8 in, 1 out]
      n174 = call "create_systemcheck_devices.vi"() -> ("error out"=w345:errorcluster)  [unwired: 11 in]
      n175 = property on="status string" class="Str"("Value"=w342) -> ()  [unwired: 2 in, 2 out]
    }
    frame #12 {
      # "not needed anymore"
      # "Create SpecObjects: load massspec info from file, create massspec objects and initialize massspecs"
      n176 = disable-structure shown="Disabled" {
        disable-tunnel: [w350 _] -> w346
        frame Disabled {
          n177 = property on="status string" class="Str"() -> ("Value"=w348:string)  [unwired: 2 in, 2 out]
          n178 = call "add_text.vi"("string in"="create spectrometers", "new string"=w348) -> ("string out"=w349:string)  [unwired: 8 in, 1 out]
          n179 = property on="status string" class="Str"("Value"=w349) -> ()  [unwired: 2 in, 2 out]
          n180 = call "create_spec_devices.vi"() -> ("error out"=w350:errorcluster)  [unwired: 11 in]
        }
        frame Enabled {
        }
      }
    }
    frame #13 {
      # "load magfield tables into each SpecObject\nmagfield tables are Objects ->MFTObj"
      n181 = call "create_MagFieldTableObjects.vi"() -> ("error out"=w351:errorcluster)  [unwired: 11 in]
      n182 = property on="status string" class="Str"() -> ("Value"=w353:string)  [unwired: 2 in, 2 out]
      n183 = call "add_text.vi"("string in"="load MagFieldTables", "new string"=w353) -> ("string out"=w352:string)  [unwired: 8 in, 1 out]
      n184 = property on="status string" class="Str"("Value"=w352) -> ()  [unwired: 2 in, 2 out]
    }
    frame #14 {
      # "read Standards.ini and create Standards objects"
      n185 = property on="status string" class="Str"() -> ("Value"=w356:string)  [unwired: 2 in, 2 out]
      n186 = call "add_text.vi"("string in"="create standards", "new string"=w356) -> ("string out"=w355:string)  [unwired: 8 in, 1 out]
      n187 = call "create_standards.vi"() -> ()  [unwired: 12 in]
      n188 = property on="status string" class="Str"("Value"=w355) -> ()  [unwired: 2 in, 2 out]
    }
    frame #15 {
      # "LoadPipettes: load pipette info from file and create pipette objects"
      n189 = property on="status string" class="Str"() -> ("Value"=w360:string)  [unwired: 2 in, 2 out]
      n190 = call "create_pipettes.vi"() -> ()  [unwired: 12 in]
      n191 = call "add_text.vi"("string in"="load pipette info", "new string"=w360) -> ("string out"=w359:string)  [unwired: 8 in, 1 out]
      n192 = property on="status string" class="Str"("Value"=w359) -> ()  [unwired: 2 in, 2 out]
    }
    frame #16 {
      # "#ConnectToDatabase"
      n193 = property on="status string" class="Str"() -> ("Value"=w362:string)  [unwired: 2 in, 2 out]
      n194 = call "add_text.vi"("string in"="not done yet!!! connect to database", "new string"=w362) -> ("string out"=w361:string)  [unwired: 8 in, 1 out]
      n195 = property on="status string" class="Str"("Value"=w361) -> ()  [unwired: 2 in, 2 out]
    }
    frame #17 {
      # "instantiate the script message object -> the object that receives \"messages\" and\nsends them to the indicator of the MainWindow"
      n196 = global read "global variables.vi" "LogFileObj"() -> (w366:refnum<class "StatusLog.lvclass">)
      n197 = global write "global variables.vi" "ScriptMsgObj"(refnum<class "Message.lvclass"> refnum ("Message.lvclass")) -> ()
      n198 = call-dynamic "add_log_entry.vi"("new entry"="instantiate script messages object", "log identifiers"="System", "StatusLog in"=w366) -> ()  [unwired: 5 in, 2 out]
    }
    frame #18 {
      # "Flag that controls whether the SampleList can proceed with\nthe next sample.\nWhen executed first the fla is on true/proceed so that the\nsample list can start"
      # "create Flags that are necessary for the operation of the software:\n\n- SampleList_proceed"
      n199 = call "FlagObjectArray_get_and_lock.vi"() -> ("FlagObjects"=w372:refnum<class "flag.lvclass">[])  [unwired: 10 in, 1 out]
      n200 = call-dynamic "Write_flag-name.vi"("flag name"="SampleList_proceed", "flag in"=refnum<class "flag.lvclass"> refnum ("flag.lvclass")) -> ("error out"=w375:errorcluster, "flag out"=w377:refnum<class "flag.lvclass">)  [unwired: 8 in]
      n201 = call-dynamic "Write_flag-state.vi"("error in (no error)"=w375, "flag state"=TRUE, "flag in"=w377) -> ("flag out"=w371:refnum<class "flag.lvclass">)  [unwired: 7 in, 1 out]
      n202 = Build Array (concatenate)(w372, w371) -> (w373:refnum<class "flag.lvclass">[])
      n203 = call "FlagObjectArray_write_and_unlock.vi"("FlagObjects"=w373) -> ()  [unwired: 10 in, 1 out]
      n204 = global read "global variables.vi" "LogFileObj"() -> (w370:refnum<class "StatusLog.lvclass">)
      n205 = call-dynamic "add_log_entry.vi"("new entry"="create flag objects", "log identifiers"="System", "StatusLog in"=w370) -> ()  [unwired: 5 in, 2 out]
    }
  }
  n206 = Merge Errors(w13, w12, w11, w10, w9, w8, w7, w6, w3, w2) -> (w5:errorcluster)
  n207 = call <vilib>:"Simple Error Handler.vi"("error source (\" \")"="MSControl startup" ("error source (\" \")"), "error in (no error)"=w5) -> ("error out"=w1:errorcluster)  [unwired: 3 in, 4 out]
  "error out" <- w1
  n208 = while {
    tunnel: w1 -> [w379]
    stop <- w381 stop-if-true
    n209 = event shown="[1] \"start button\": Value Change" {
      selector: _ -> [_ _ _]
      dyn-events: _ -> [_ _ _]
      timeout: 1000 -> [_ _ _]
      tunnel: [w382 FALSE FALSE] -> w381
      tunnel: w379 -> [_ _ _]
      event Timeout {
        n210 = event-data() -> ()  [unwired: 1 in, 3 out]
        n211 = global read "global variables.vi" "close prog flag"() -> (w382:bool)
        n212 = case shown="True" w382 {
          frame False {
          }
          frame True {
            n213 = invoke class="VI" method="FP.Close"() -> ()  [unwired: 3 in, 3 out]
          }
        }
      }
      event "start button": Value Change {
        w383 = FALSE ("Visible")
        # "don't stop loop.\nif VI stops all the queues are being destroyed"
        n214 = event-data() -> ()  [unwired: 1 in, 6 out]
        n215 = stacked-sequence {
          frame #0 {
            # "go through all switch controller objects, initialize, read IDs and read current switch states"
            n216 = call "InstrumentObjectArray_get_and_lock.vi"() -> ("InstrumentsObjects"=w385:refnum<class "instrument.lvclass">[])  [unwired: 10 in, 1 out]
            n217 = for {
              tunnel: w385 -> [w389] mode=indexing
              tunnel: [w388] -> w386 mode=indexing
              tunnel: [w387] -> _
              n218 = while {
                tunnel: w389 -> [w400]
                tunnel: [w396] -> w388
                tunnel: [w391] -> w387
                stop <- w395 stop-if-true
                n219 = call-dynamic "Read_name.vi"("instrument in"=w400) -> ("error out"=w403:errorcluster, "name"=w394:string, "instrument out"=w404:refnum<class "instrument.lvclass">)  [unwired: 8 in]
                n220 = call-dynamic "initialize.vi"("error in (no error)"=w403, "instrument in"=w404) -> ("error out"=w391:errorcluster, "String outout"=w390:string, "initialized?"=w397:bool, "instrument out"=w402:refnum<class "instrument.lvclass">)  [unwired: 6 in]
                n221 = case shown="True" w397 {
                  tunnel: w402 -> [w416 w431]
                  tunnel: w391 -> [_ w429]
                  tunnel: [w415 w427] -> w396
                  tunnel: [w410 TRUE] -> w395
                  tunnel: w394 -> [w407 _]
                  tunnel: [_ w426] -> _
                  frame False {
                    n222 = Format Into String(initial string="Unable to find Instrument: %s" ("message"), w407) -> (resulting string=w408:string)  [unwired: 2 in, 1 out]
                    n223 = call <vilib>:"Three Button Dialog.vi"("Right Button Text (\"Cancel\")"="Retry" ("Right Button Text (\"Cancel\")"), "Center Button Text (\"No\")"="Quit" ("F button name (\"Cancel\")"), "Left Button Text (\"Yes\")"="Proceed without" ("T button name (\"OK\")"), "message"=w408) -> ("Which Button?"=w414:T10)  [unwired: 7 in]
                    n224 = case shown="\"Right Button\"" w414 {
                      tunnel: w416 -> [w420 w422 w425]
                      tunnel: [w419 w422 w425] -> w415
                      tunnel: [TRUE TRUE FALSE] -> w410
                      frame "Left Button", Default {
                        n225 = call-dynamic "Write_available.vi"("available?"=FALSE, "instrument in"=w420) -> ("instrument out"=w419:refnum<class "instrument.lvclass">)  [unwired: 8 in, 1 out]
                      }
                      frame "Center Button" {
                        n226 = Stop(stop? (T)=TRUE) -> ()
                      }
                      frame "Right Button" {
                        # "Retry"
                      }
                    }
                  }
                  frame True {
                    w434 = u16 1 items=["local", "remote", "remot with lock-out"] ("mode")
                    n227 = call-dynamic "Write_available.vi"("error in (no error)"=w429, "available?"=TRUE, "instrument in"=w431) -> ("error out"=w428:errorcluster, "instrument out"=w430:refnum<class "instrument.lvclass">)  [unwired: 7 in]
                    n228 = call-dynamic "set_remote-interface-mode.vi"("error in (no error)"=w428, "mode"=w434, "instrument in"=w430) -> ("error out"=w426:errorcluster, "instrument out"=w427:refnum<class "instrument.lvclass">)  [unwired: 7 in]
                  }
                }
                n229 = Unbundle By Name(w391) -> ("code"=w393:i32)
                n230 = Format Into String(format string="init Instr: %s, ErrorCode=%d, Answer: %s", w394, w393, w390) -> (resulting string=w392:string)  [unwired: 2 in, 1 out]
                n231 = property on="status string" class="Str"() -> ("Value"=w406:string)  [unwired: 2 in, 2 out]
                n232 = global read "global variables.vi" "LogFileObj"() -> (w401:refnum<class "StatusLog.lvclass">)
                n233 = call "add_text.vi"("string in"=w392, "new string"=w406) -> ("string out"=w405:string)  [unwired: 8 in, 1 out]
                n234 = property on="status string" class="Str"("Value"=w405) -> ()  [unwired: 2 in, 2 out]
                n235 = call-dynamic "add_log_entry.vi"("new entry"=w392, "log identifiers"="Instrument Object", "StatusLog in"=w401) -> ()  [unwired: 5 in, 2 out]
              }
            }
            n236 = call "InstrumentObjectArray_write_and_unlock.vi"("InstrumentObjects"=w386) -> ()  [unwired: 10 in, 1 out]
          }
          frame #1 {
            # "go through every SwitchObject and compare the default state with the actual state of the switch"
            n237 = call "PrepLineObjectArray_get_and_lock_queue.vi"() -> ("PrepLineObjects"=w435:refnum<class "PrepLineObject.lvclass">[])  [unwired: 10 in, 1 out]
            n238 = for {
              tunnel: w435 -> [w440] mode=indexing
              tunnel: [w437] -> w436 mode=indexing
              n239 = call-dynamic "Read_type.vi"("PrepLinePictureObjects in"=w440) -> ("type"=w438:string, "PrepLinePictureObjects out"=w439:refnum<class "PrepLineObject.lvclass">)  [unwired: 8 in, 1 out]
              n240 = case shown="\"switch\"" w438 {
                tunnel: w439 -> [w441 w446]
                tunnel: [w441 w448] -> w437
                frame "False", Default {
                }
                frame "switch" {
                  # "still the\ndefault\nvalue"
                  n241 = call-dynamic "Read_instrument-object.vi"("PrepLineObject in"=w446) -> ("instrument.lvclass"=w445:refnum<class "instrument.lvclass">)  [unwired: 8 in, 2 out]
                  n242 = call-dynamic "Read_instrument.vi"("PrepLinePictureObjects in"=w446) -> ("error out"=w443:errorcluster)  [unwired: 7 in, 2 out]
                  n243 = call-dynamic "Read_channel.vi"("PrepLineObject in"=w446) -> ("channel"=w453:u16)  [unwired: 8 in, 2 out]
                  n244 = call-dynamic "Read_state.vi"("PrepLineObject in"=w446) -> ("state"=w451:bool, "PrepLineObject out"=w449:refnum<class "PrepLineObject.lvclass">)  [unwired: 8 in, 1 out]
                  n245 = call-dynamic "get_switch.vi"("error in (no error)"=w443, "channel"=w453, "instrument in"=w445) -> ("error out"=w444:errorcluster, "String"=w442:string, "actual switch state"=w452:bool, "instrument out"=w447:refnum<class "instrument.lvclass">)  [unwired: 5 in]
                  n246 = Equal?(x=w452, y=w451) -> (x = y?=w450:bool)
                  n247 = case shown="False" w450 {
                    tunnel: w449 -> [w456 w477]
                    tunnel: [w459 w477] -> w448
                    tunnel: w447 -> [w458 _]
                    tunnel: w444 -> [_ _]
                    tunnel: w442 -> [_ _]
                    frame False {
                      # "it's not in default"
                      n248 = call-dynamic "Read_instrument.vi"("PrepLinePictureObjects in"=w456) -> ("instrument name"=w462:string)  [unwired: 7 in, 2 out]
                      n249 = call-dynamic "Read_channel.vi"("PrepLineObject in"=w456) -> ("channel"=w457:u16)  [unwired: 8 in, 2 out]
                      n250 = call-dynamic "Read_state.vi"("PrepLineObject in"=w456) -> ("state"=w455:bool, "PrepLineObject out"=w454:refnum<class "PrepLineObject.lvclass">)  [unwired: 8 in, 1 out]
                      n251 = Format Into String(format string="Switch channel %d\nof %s\nis not in default state.\nSwitch?", w457, w462) -> (resulting string=w461:string)  [unwired: 2 in, 1 out]
                      n252 = Two Button Dialog(message=w461) -> (T button?=w460:bool)  [unwired: 2 in]
                      n253 = case shown="False" w460 {
                        tunnel: [w466 w473] -> w459
                        tunnel: w458 -> [_ w476]
                        tunnel: w457 -> [_ w475]
                        tunnel: w455 -> [w465 w471]
                        tunnel: w454 -> [w467 w474]
                        frame False {
                          # "don't switch to default\n-> change state"
                          n254 = Not(x=w465) -> (.not. x?=w464:bool)
                          n255 = call-dynamic "Write_state.vi"("state"=w464, "PrepLineObject in"=w467) -> ("PrepLineObject out"=w466:refnum<class "PrepLineObject.lvclass">)  [unwired: 8 in, 1 out]
                        }
                        frame True {
                          # "switch to default"
                          n256 = global read "global variables.vi" "LogFileObj"() -> (w470:refnum<class "StatusLog.lvclass">)
                          n257 = call-dynamic "set switch.vi"("state"=w471, "channel"=w475, "instrument in"=w476) -> ("error out"=w472:errorcluster)  [unwired: 7 in, 1 out]
                          n258 = call-dynamic "Write_state.vi"("error in (no error)"=w472, "state"=w471, "PrepLineObject in"=w474) -> ("PrepLineObject out"=w473:refnum<class "PrepLineObject.lvclass">)  [unwired: 7 in, 1 out]
                          n259 = call-dynamic "add_log_entry.vi"("new entry"="set switch to default", "log identifiers"="Instrument Object", "StatusLog in"=w470) -> ()  [unwired: 5 in, 2 out]
                        }
                      }
                    }
                    frame True {
                      # "it's in default already"
                    }
                  }
                }
              }
            }
            n260 = call "PrepLineObjectArray_write_and_unlock_queue.vi"("PrepLineObjArray"=w436) -> ()  [unwired: 10 in, 1 out]
          }
          frame #2 {
            # "there's a problem with queues.\n\nWhen loading those windows dynamically\nthey loose the queues that are generated by this VI.\nNot sure why.\n\nDon't close this VI"
            # "open main windows dynamically"
            n261 = call "open_MainWindow_dyn.vi"() -> ()  [unwired: 11 in, 1 out]
            n262 = call "open_PrepLine_window_dyn.vi"() -> ()  [unwired: 11 in, 1 out]
            n263 = call "open_status_window_dyn.vi"() -> ()  [unwired: 11 in, 1 out]
            n264 = property on="status string" class="Str"() -> ("Value"=w479:string)  [unwired: 2 in, 2 out]
            n265 = call "add_text.vi"("string in"="open main widnows", "new string"=w479) -> ("string out"=w478:string)  [unwired: 8 in, 1 out]
            n266 = property on="status string" class="Str"("Value"=w478) -> ()  [unwired: 2 in, 2 out]
            n267 = global read "global variables.vi" "LogFileObj"() -> (w483:refnum<class "StatusLog.lvclass">)
            n268 = call-dynamic "add_log_entry.vi"("new entry"="Open main window, PrepLineWindow and Status window\n\n=== startup completed ===\n", "log identifiers"="System", "StatusLog in"=w483) -> ()  [unwired: 5 in, 2 out]
          }
          frame #3 {
            # "minimize the frotpanel of this VI"
            n269 = property class="VI"("FP.State"=T9."Minimized" ("Front Panel Window:State")) -> ()  [unwired: 2 in, 2 out]
            n270 = Wait (ms)(milliseconds to wait=u32 2000) -> ()  [unwired: 1 out]
            n271 = Request Deallocation(TRUE ("flag")) -> ()
          }
        }
        n272 = property on="start button" class="Bool (strict)"("Visible"=w383) -> ()  [unwired: 2 in, 2 out]
        n273 = property on="setup button" class="Bool (strict)"("Visible"=w383) -> ()  [unwired: 2 in, 2 out]
      }
      event "setup button": Mouse Down? {
        w489 = TRUE ("Visible")
        # "#SetupButton finish the setup UI that shows all setup data"
        n274 = event-data() -> ()  [unwired: 1 in, 8 out]
        n275 = call "setup_window.vi"() -> ()  [unwired: 12 in]
        n276 = property on="start button" class="Bool (strict)"("Visible"=w489) -> ()  [unwired: 2 in, 2 out]
        n277 = property on="setup button" class="Bool (strict)"("Visible"=w489) -> ()  [unwired: 2 in, 2 out]
        n278 = event-data("Discard?"=TRUE) -> ()  [unwired: 1 in, 1 out]
      }
    }
  }
